vi "General VISA Transactions.vi"(4 "Error In":errorcluster, 5 "Array":string[](array[string]), 7 "Open VISA Resource name":refnum<visa-resource-name>) -> (0 "Error Out":errorcluster, 1 "Measurement":dbl[](array[numeric]), 2 "Variant":variant, 3 "dup VISA session":refnum<visa-resource-name>)   [LabVIEW 2021]
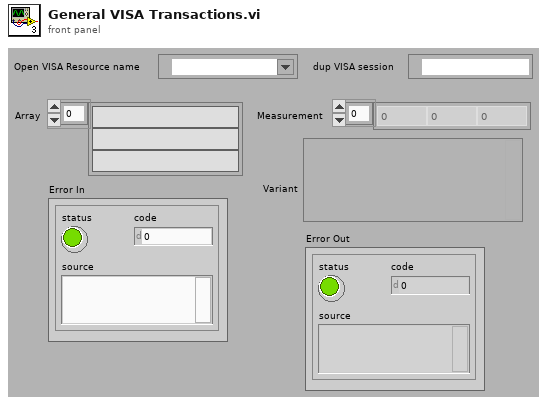
[diagram p1: front panel]
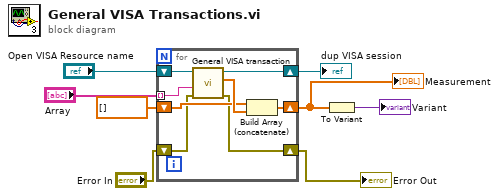
[diagram p0: block diagram]
diagram:
  n1 = for {
    tunnel: "Array" -> [w16] mode=indexing
    shift-right: [w15] -> w7
    shift-left: "Open VISA Resource name" -> [w14]
    shift-right: [w12] -> w4
    shift-left: dbl[] [] ("Measurement") -> [w11]
    shift-right: [w10] -> w1
    shift-left: "Error In" -> [w9]
    n2 = call "General VISA transaction.vi"("error in (no error)"=w9, "Command String"=w16, "VISA Session"=w14) -> ("error out"=w10:errorcluster, "Measurement"=w13:dbl[], "dup VISA Session"=w15:refnum<visa-resource-name>)  [unwired: 3 in, 3 out]
    n3 = Build Array (concatenate)(w11, w13) -> (w12:dbl[])
  }
  "dup VISA session" <- w7
  "Measurement" <- w4
  "Error Out" <- w1
  n4 = To Variant(anything=w4) -> (Variant=→"Variant":variant)
